vi "Size.vi"(8 "error in (no error)":errorcluster, 11 "String Array in":refnum<class "String Array.lvclass">) -> (0 "error out":errorcluster, 2 "Size":i32, 3 "String Array out":refnum<class "String Array.lvclass">)   [LabVIEW 2020, in "Data.lvlib" / "String Array.lvclass"]
doc: "Return the size of the generic data element."
uses:
  String Array.lvclass
  String Array.lvclass/String Array.ctl
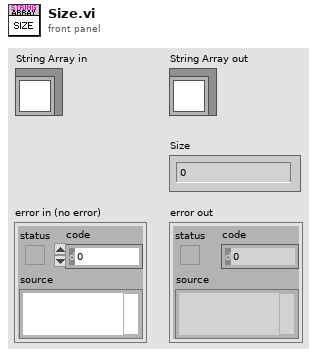
[diagram p1: front panel]
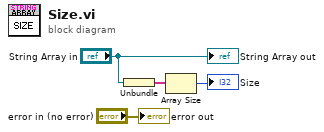
[diagram p0: block diagram]
diagram:
  n1 = Unbundle("String Array in") -> (w2:string[])
  n2 = Array Size(array=w2) -> (size(s)=→"Size":i32)
  "error out" <- "error in (no error)"
  "String Array out" <- "String Array in"
